vi "test harness_FXP_L_ye_Bend_u_singleAxis.vi"(8 "error in (no error)":errorcluster, 11 "TestCase in":refnum<class "FXP_observer_TestCase.lvclass">) -> (0 "error out":errorcluster, 3 "TestCase out":refnum<class "FXP_observer_TestCase.lvclass">)   [LabVIEW 2017, in "FXP_observer_TestCase.lvclass"]
uses:
  FXP_observer_TestCase.lvclass
  <vilib>/rvi/DesktopExecutionNode/Execution/niFpgaDEN_Execute.vi
  <vilib>/rvi/DesktopExecutionNode/DesktopExecutionNode.xnode
  <vilib>/addons/_JKI Toolkits/VI Tester/TestCase.llb/TestCase.lvclass
  C:/Program Files (x86)/National Instruments/LabVIEW 2017/vi.lib/addons/_JKI Toolkits/VI Tester/TestCase.llb/TestCase.lvclass
panel:
  out "xk_1_2":fxp<+/-,32,5>[](array[numeric])
  out "x+y":fxp<+/-,51,11>[](array[numeric])
  out "xk_1_1":fxp<+/-,32,5>[](array[numeric])
  out "error (x_1_1)":errorcluster
  out "error (xu)":errorcluster
  out "error (yd)":errorcluster
  in  "Bz":fxp<+/-,32,5>[](array[numeric])=[1.0, 0.5, 0.20000000298023224, 0.20000000298023224, 0.29999999701976776, 2.0, 0.0, 0.0, 0.0, 0.0, 0.0, 0.0, 0.0, 0.0, 0.0, 0.0, 0.0, 0.0, 0.0, 0.0, 0.0, 0.0, 0.0, 0.0, 0.0, 0.0, 0.0, 0.0, 0.0, 0.0, 0.0, 0.0, 0.0, 0.0, 0.0, 0.0, 0.0, 0.0, 0.0, 0.0, 0.0, 0.0, 0.0, 0.0, 0.0, 0.0, 0.0, 0.0, 0.0, 0.0]
  in  "U(k): ux":fxp<+/-,18,5>=0.14501953125
  in  "y(k)":fxp<+/-,18,5>=0.123046875
  in  "NS":u8=6
  in  "Ldist":fxp<+/-,32,5>[](array[numeric])=[1.0, 0.5, 0.20000000298023224, 0.20000000298023224, 0.29999999701976776, 2.0, 0.0, 0.0, 0.0, 0.0, 0.0, 0.0, 0.0, 0.0, 0.0, 0.0, 0.0, 0.0, 0.0, 0.0, 0.0, 0.0, 0.0, 0.0, 0.0, 0.0, 0.0, 0.0, 0.0, 0.0, 0.0, 0.0, 0.0, 0.0, 0.0, 0.0, 0.0, 0.0, 0.0, 0.0, 0.0, 0.0, 0.0, 0.0, 0.0, 0.0, 0.0, 0.0, 0.0, 0.0]
  in  "x":fxp<+/-,32,5>[](array[numeric])=[1.0, 2.0, 3.0, 4.0, 5.0, 2.0, 0.0, 0.0, 0.0, 0.0, 0.0, 0.0, 0.0, 0.0, 0.0, 0.0, 0.0, 0.0, 0.0, 0.0, 0.0, 0.0, 0.0, 0.0, 0.0, 0.0, 0.0, 0.0, 0.0, 0.0, 0.0, 0.0, 0.0, 0.0, 0.0, 0.0, 0.0, 0.0, 0.0, 0.0, 0.0, 0.0, 0.0, 0.0, 0.0, 0.0, 0.0, 0.0, 0.0, 0.0]
  # "Remember that Ldist and Bz only have\ntwo integer bits!"
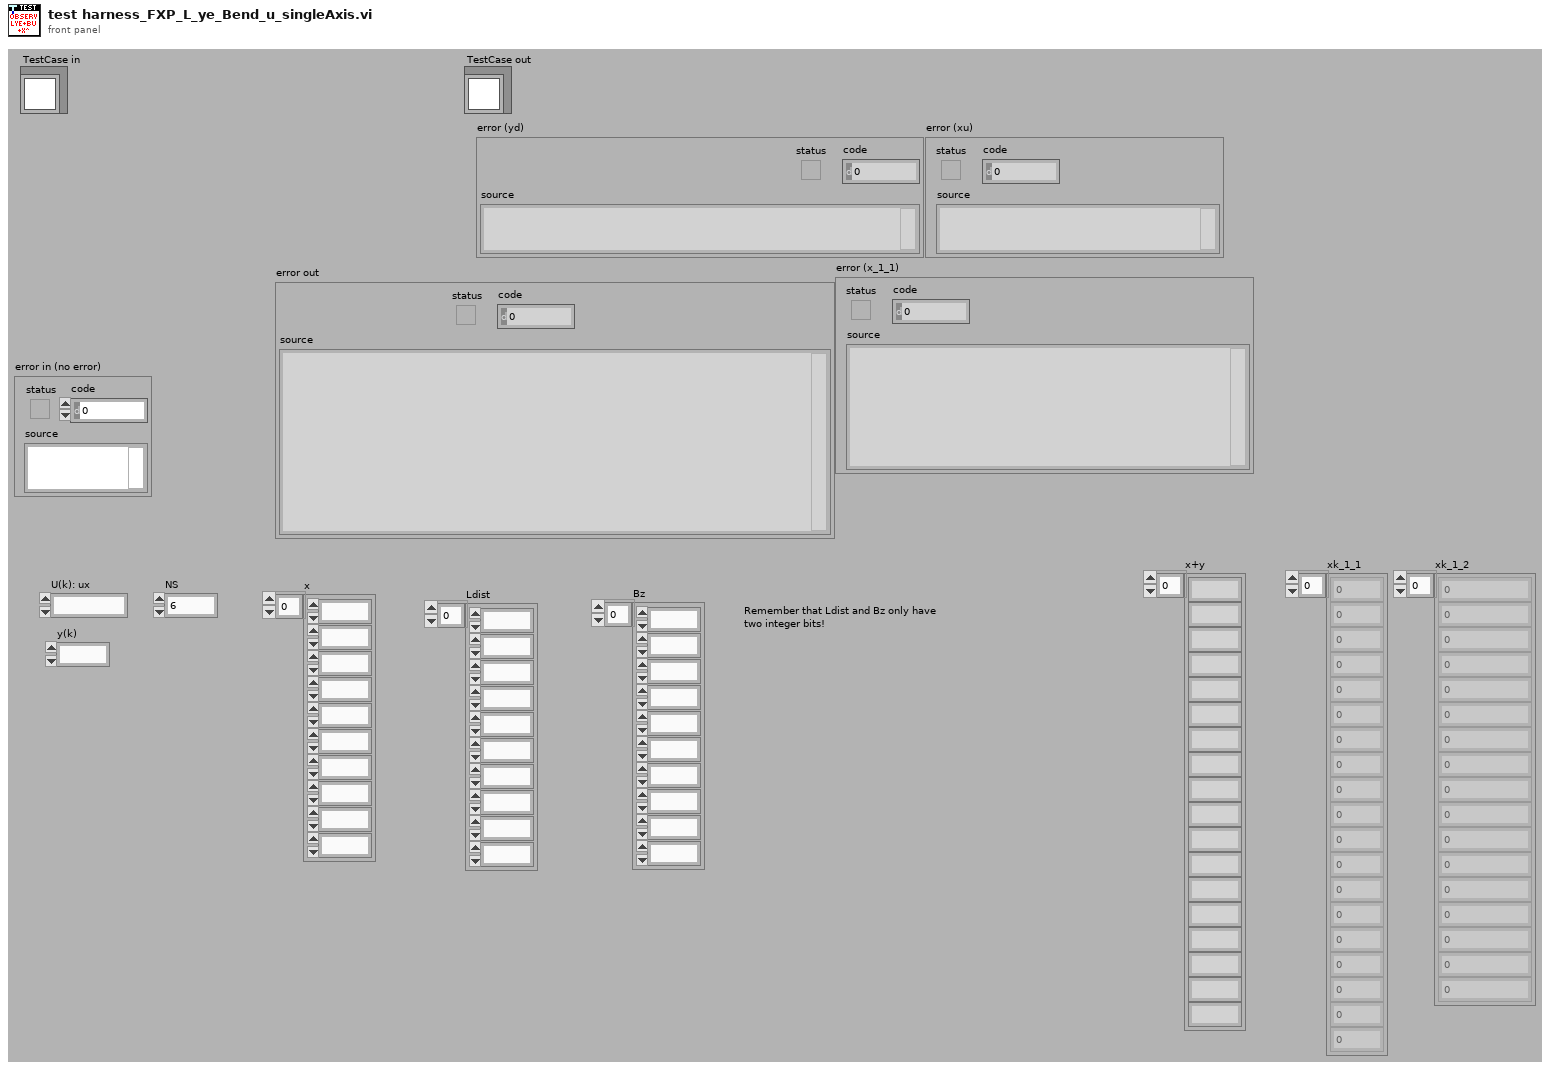
[diagram p1: front panel]
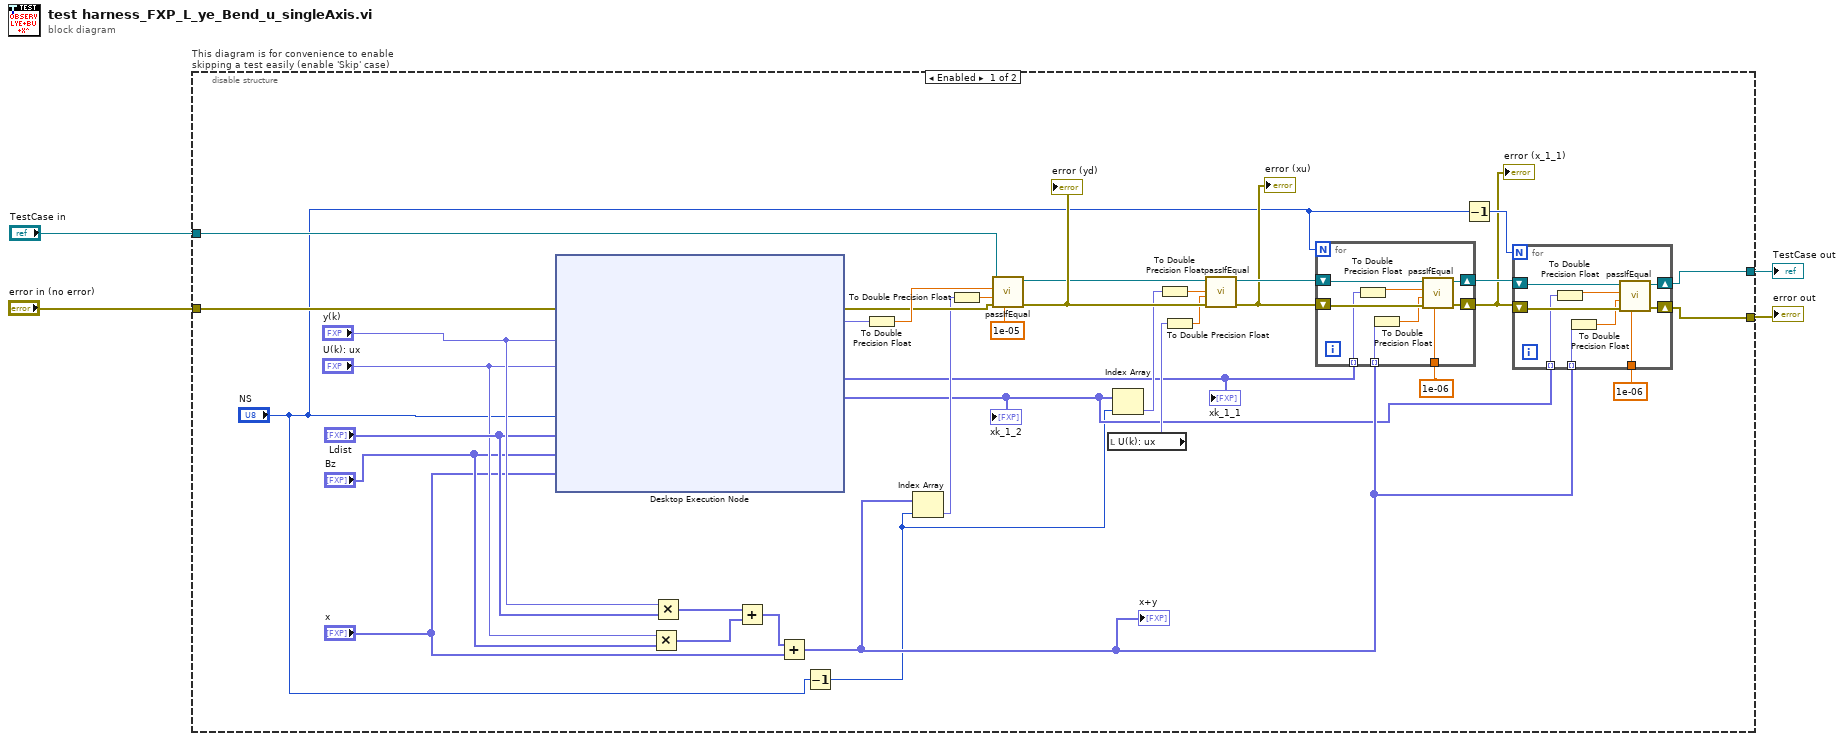
[diagram p0: block diagram]
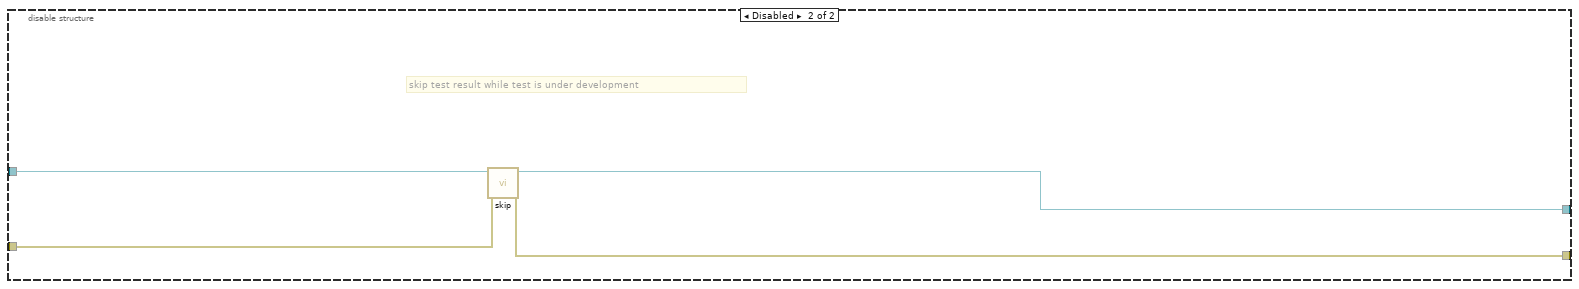
[diagram p2: hidden frame]
diagram:
  n1 = disable-structure "This diagram is for convenience to enable skipping a test easily (enable 'Skip' case)" shown="Enabled" {
    disable-tunnel: "TestCase in" -> [w40 w62]
    disable-tunnel: [w14 w60] -> w1
    disable-tunnel: [w13 w61] -> w3
    disable-tunnel: "error in (no error)" -> [w36 w59]
    frame Enabled {
      n2 = xnode "Desktop Execution Node"("Error In"=w36, "y(k)"="y(k)", "U(k): ux"="U(k): ux", "NS"="NS", "Ldist"="Ldist", "Bz"="Bz", "x"="x") -> ("Error Out"=w37:errorcluster, "yd_est"=w27:fxp<+/-,32,5>, "xk_1_1"=w17:fxp<+/-,32,5>[], "xk_1_2"=w9:fxp<+/-,32,5>[])
      "xk_1_1" <- w17
      "xk_1_2" <- w9
      n3 = Multiply(x="U(k): ux", y="Bz") -> (x*y=w30:fxp<+/-,50,10>[])
      n4 = Multiply(x="y(k)", y="Ldist") -> (x*y=w31:fxp<+/-,50,10>[])
      n5 = Add(x=w31, y=w30) -> (x+y=w29:fxp<+/-,51,11>[])
      n6 = Add(x=w29, y="x") -> (x+y=w10:fxp<+/-,51,11>[])
      "x+y" <- w10
      n7 = Decrement(x="NS") -> (x-1=w5:u8)
      n8 = To Double Precision Float(number=w27) -> (double precision float=w38:dbl)
      n9 = Index Array(array=w10, index=w5) -> (element=w25:fxp<+/-,51,11>)
      n10 = To Double Precision Float(number=w25) -> (double precision float=w26:dbl)
      n11 = call-dynamic "passIfEqual.vi"("delta (optional)"=1e-05 ("del u_x"), "error in (no error)"=w37, "y"=w26, "x"=w38, "TestCase in"=w40) -> ("error out"=w24:errorcluster, "TestCase out"=w23:refnum<class "FXP_observer_TestCase.lvclass">)  [unwired: 5 in]
      "error (yd)" <- w24
      n12 = local read "U(k): ux"() -> (w19:fxp<+/-,18,5>)
      n13 = Index Array(array=w9, index=w5) -> (element=w21:fxp<+/-,32,5>)
      n14 = To Double Precision Float(number=w21) -> (double precision float=w22:dbl)
      n15 = To Double Precision Float(number=w19) -> (double precision float=w20:dbl)
      n16 = call-dynamic "passIfEqual.vi"("error in (no error)"=w24, "y"=w20, "x"=w22, "TestCase in"=w23) -> ("error out"=w8:errorcluster, "TestCase out"=w18:refnum<class "FXP_observer_TestCase.lvclass">)  [unwired: 6 in]
      "error (xu)" <- w8
      n17 = for {
        N: "NS" -> [_]
        shift-right: [w58] -> w15
        shift-left: w18 -> [w55]
        shift-right: [w57] -> w7
        shift-left: w8 -> [w56]
        tunnel: w10 -> [w54] mode=indexing
        tunnel: w17 -> [w51] mode=indexing
        tunnel: 1e-06 ("del u_x") -> [w50]
        n18 = To Double Precision Float(number=w51) -> (double precision float=w52:dbl)
        n19 = To Double Precision Float(number=w54) -> (double precision float=w53:dbl)
        n20 = call-dynamic "passIfEqual.vi"("delta (optional)"=w50, "error in (no error)"=w56, "y"=w53, "x"=w52, "TestCase in"=w55) -> ("error out"=w57:errorcluster, "TestCase out"=w58:refnum<class "FXP_observer_TestCase.lvclass">)  [unwired: 5 in]
      }
      "error (x_1_1)" <- w7
      n21 = Decrement(x="NS") -> (x-1=w11:u8)
      n22 = for {
        N: w11 -> [_]
        shift-right: [w49] -> w14
        shift-left: w15 -> [w46]
        shift-right: [w48] -> w13
        shift-left: w7 -> [w47]
        tunnel: w10 -> [w45] mode=indexing
        tunnel: w9 -> [w42] mode=indexing
        tunnel: 1e-06 ("del u_x") -> [w41]
        n23 = To Double Precision Float(number=w42) -> (double precision float=w43:dbl)
        n24 = To Double Precision Float(number=w45) -> (double precision float=w44:dbl)
        n25 = call-dynamic "passIfEqual.vi"("delta (optional)"=w41, "error in (no error)"=w47, "y"=w44, "x"=w43, "TestCase in"=w46) -> ("error out"=w48:errorcluster, "TestCase out"=w49:refnum<class "FXP_observer_TestCase.lvclass">)  [unwired: 5 in]
      }
    }
    frame Disabled {
      # "skip test result while test is under development"
      n26 = call <vilib>:"skip.vi"("error in (no error)"=w59, "TestCase in"=w62) -> ("error out"=w61:errorcluster, "TestCase out"=w60:refnum<class "FXP_observer_TestCase.lvclass">)  [unwired: 8 in]
    }
  }
  "error out" <- w3
  "TestCase out" <- w1
